vi "SPTI Read10 Command.vi"(8 "error in (no error)":errorcluster, 9 "Block Size (512)":u32=512, 10 "Nr Blocks":u32=1, 11 "Start LBA":u32 format="%x") -> (0 "error out":errorcluster, 3 "Read Data":u8[](array[numeric]) format="%02x")   [LabVIEW 2014]
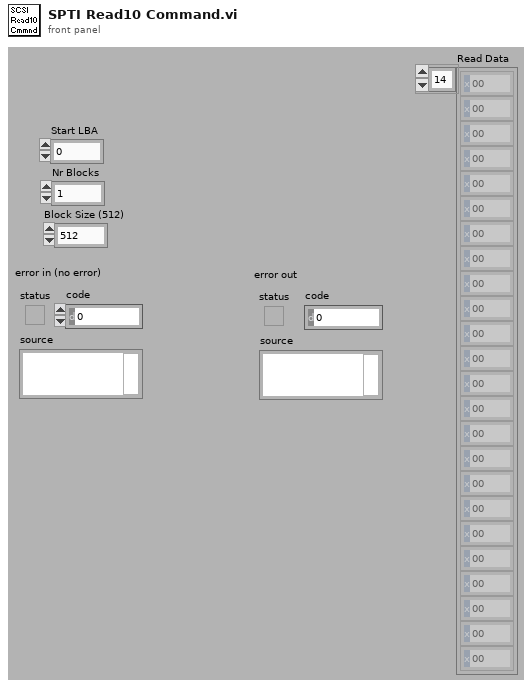
[diagram p1: front panel]
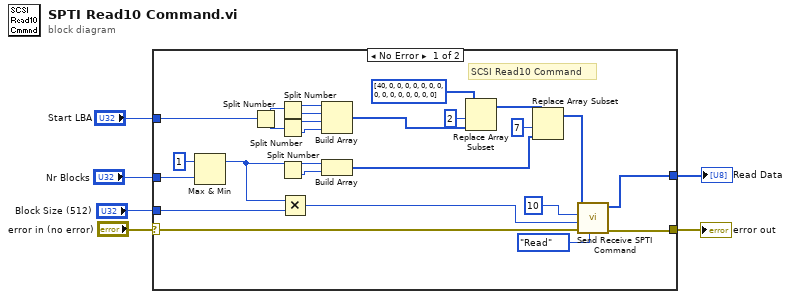
[diagram p0: block diagram]
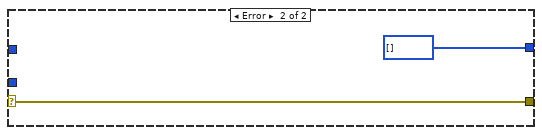
[diagram p2: hidden frame]
diagram:
  n1 = case shown="No Error" "error in (no error)" {
    selector: "error in (no error)" -> [w32 w34]
    tunnel: [w29 w34] -> w5
    tunnel: "Start LBA" -> [w28 _]
    tunnel: "Nr Blocks" -> [w18 _]
    tunnel: "Block Size (512)" -> [w19 _]
    tunnel: [w14 u8[] [] ("Received Data")] -> w1
    frame No Error {
      # "SCSI Read10 Command"
      n2 = Max & Min(x=u32 1, y=w18) -> (max(x,y)=w9:u32)  [unwired: 1 out]
      n3 = Split Number(x=w28) -> (hi(x)=w27:u16, lo(x)=w26:u16)
      n4 = Split Number(x=w27) -> (hi(x)=w25:u8, lo(x)=w24:u8)
      n5 = Split Number(x=w26) -> (hi(x)=w23:u8, lo(x)=w22:u8)
      n6 = Split Number(x=w9) -> (hi(x)=w20:u16, lo(x)=w21:u16)
      n7 = Multiply(x=w9, y=w19) -> (x*y=w17:u32)
      n8 = Build Array(w25, w24, w23, w22) -> (w12:u8[])
      n9 = Build Array(w20, w21) -> (w8:u16[])
      n10 = Replace Array Subset(array=u8[] [40, 0, 0, 0, 0, 0, 0, 0, 0, 0, 0, 0, 0, 0, 0, 0] ("Command Data Block"), new element=w12, index=2) -> (w11:u8[])
      n11 = Replace Array Subset(array=w11, new element=w8, index=7) -> (w7:u8[])
      n12 = call "Send Receive SPTI Command.vi"("read/write"=enum16{"Read", "Write"}."Read", "error in (no error)"=w32, "Expected Nr Response Bytes"=w17, "Valid CDB bytes"=u8 10, "Command Data Block"=w7) -> ("error out"=w29:errorcluster, "Received Data"=w14:u8[])  [unwired: 5 in]
    }
    frame Error {
    }
  }
  "error out" <- w5
  "Read Data" <- w1
